vi "MRayComputeDistanc.vi"(8 "Y Image Resolution":i32, 9 "X Image Resolution":i32, 10 "Bounding Box":T1) -> (2 "Target Center (-1 to 1)":cluster{"X":dbl, "Y":dbl}, 3 "Distance (ft)":dbl)   [LabVIEW 2011]
panel:
  in  "Vision Angle":i32=47
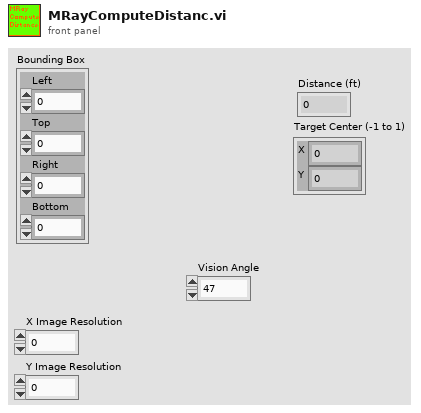
[diagram p1: front panel]
types:
  T1 = cluster{"Left":dbl, "Top":dbl, "Right":dbl, "Bottom":dbl}
  T2 = cluster{"X Image Resolution":i32, "Y Image Resolution":i32}
  T3 = cluster{"X Image Resolution":dbl, "Y Image Resolution":dbl}
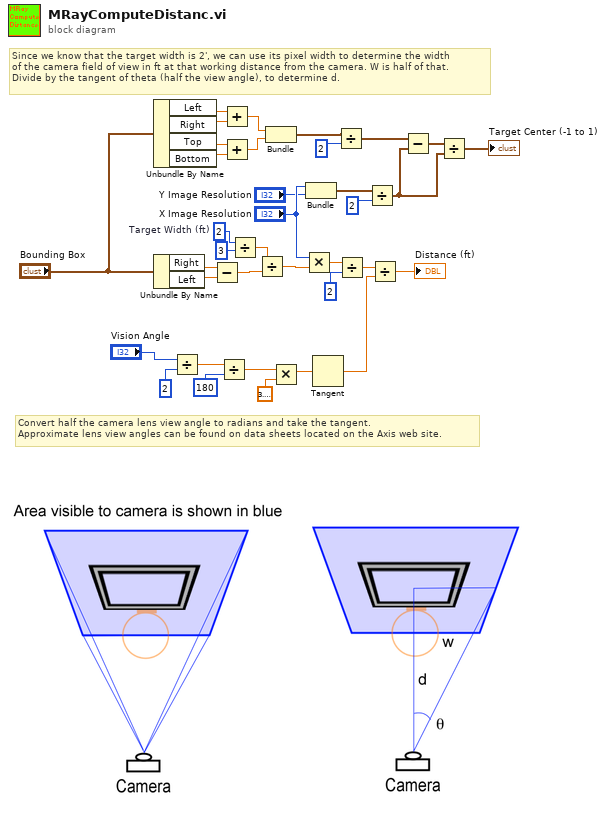
[diagram p0: block diagram]
diagram:
  w3 = 2  # Target Width (ft)
  # "Convert half the camera lens view angle to radians and take the tangent.\nApproximate lens view angles can be found on data sheets located on the Axis web site."
  # "Since we know that the target width is 2', we can use its pixel width to determine the width\nof the camera field of view in ft at that working distance from the camera. W is half of that.\nDivide by the tangent of theta (half the view angle), to determine d."
  n1 = Unbundle By Name("Bounding Box") -> ("Left"=w19:dbl, "Right"=w20:dbl, "Top"=w22:dbl, "Bottom"=w21:dbl)
  n2 = Unbundle By Name("Bounding Box") -> ("Right"=w27:dbl, "Left"=w26:dbl)
  n3 = Divide(x="Vision Angle", y=2) -> (x/y=w33:dbl)
  n4 = Subtract(x=w27, y=w26) -> (x-y=w25:dbl)
  n5 = Divide(x=w33, y=180) -> (x/y=w32:dbl)
  n6 = Add(x=w19, y=w20) -> (x+y=w17:dbl)
  n7 = Add(x=w22, y=w21) -> (x+y=w16:dbl)
  n8 = Divide(x=w3, y=3) -> (x/y=w1:dbl)
  n9 = Divide(x=w1, y=w25) -> (x/y=w24:dbl)
  n10 = Bundle(w17, w16) -> (w11:cluster{dbl, dbl})  [unwired: 1 in]
  n11 = Multiply(x=w32, y=3.141592653589793) -> (x*y=w6:dbl)
  n12 = Multiply(x="X Image Resolution", y=w24) -> (x*y=w28:dbl)
  n13 = Bundle("X Image Resolution"="X Image Resolution", "Y Image Resolution"="Y Image Resolution") -> (w13:T2)  [unwired: 1 in]
  n14 = Tangent(1:w6) -> (0:w36:dbl)
  n15 = Divide(x=w11, y=2) -> (x/y=w10:cluster{dbl, dbl})
  n16 = Divide(x=w28, y=2) -> (x/y=w30:dbl)
  n17 = Divide(x=w13, y=2) -> (x/y=w8:T3)
  n18 = Divide(x=w30, y=w36) -> (x/y=→"Distance (ft)":dbl)
  n19 = Subtract(x=w10, y=w8) -> (x-y=w9:cluster{dbl, dbl})
  n20 = Divide(x=w9, y=w8) -> (x/y=→"Target Center (-1 to 1)":cluster{dbl, dbl})
